vi "Attenuator_AbsMove.vi"(3 "error in (no error)":errorcluster caption="错误输入（无错误）", 4 "Position":i32, 5 "Axis":u16) -> (0 "error out":errorcluster)   [LabVIEW 2018]
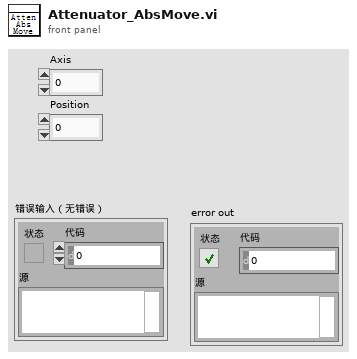
[diagram p1: front panel]
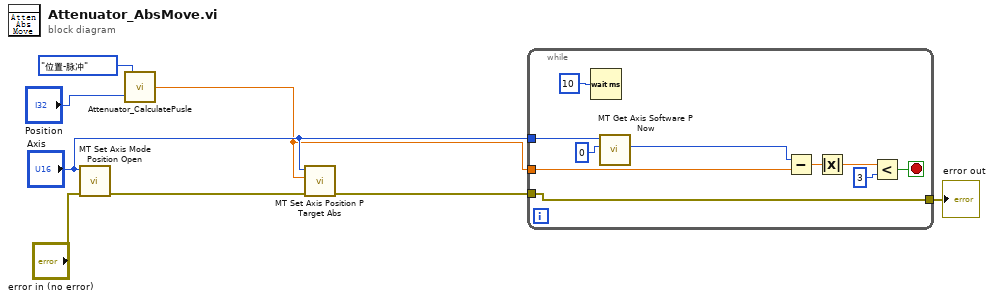
[diagram p0: block diagram]
diagram:
  n1 = call "MT Set Axis Mode Position Open.vi"("error in (no error)"="error in (no error)", "AObj"="Axis") -> ("error out"=w8:errorcluster)  [unwired: 8 in, 1 out]
  n2 = call "Attenuator_CalculatePusle.vi"("计算状态"=enum32{"位置-脉冲", "脉冲-位置"}."位置-脉冲", "数据"="Position") -> ("dataout"=w2:dbl)  [unwired: 2 in]
  n3 = call "MT Set Axis Position P Target Abs.vi"("error in (no error)"=w8, "Value"=w2, "AObj"="Axis") -> ("error out"=w7:errorcluster)  [unwired: 7 in, 1 out]
  n4 = while {
    tunnel: w7 -> [w9]
    tunnel: "Axis" -> [w18]
    tunnel: w2 -> [w15]
    tunnel: [w9] -> w5
    stop <- w11 stop-if-true
    n5 = Wait (ms)(milliseconds to wait=u32 10 ("等待时间（毫秒）")) -> ()  [unwired: 1 out]
    n6 = call "MT Get Axis Software P Now.vi"("pValue"=0, "AObj"=w18) -> ("pValue out"=w16:i32)  [unwired: 7 in, 2 out]
    n7 = Subtract(x=w16, y=w15) -> (x-y=w14:dbl)
    n8 = Absolute Value(x=w14) -> (abs(x)=w13:dbl)
    n9 = Less?(x=w13, y=3) -> (x < y?=w11:bool)
  }
  "error out" <- w5
